vi "Multiple Event Registration1.vi"(11 "Test Case In":refnum<class "Tests Event MessengerM.lvclass">) -> (0 "error out":errorcluster, 3 "Test Case Out":refnum<class "Tests Event MessengerM.lvclass">)   [LabVIEW 2020, in "Tests Event MessengerM.lvclass"]
uses:
  Tests Event MessengerM.lvclass
  C:/Program Files/National Instruments/LabVIEW 2026/vi.lib/Astemes/LUnit/Test Case.lvclass
  <vilib>/Astemes/LUnit/Test Case.lvclass/Test Case.ctl
  4993e8ee-a06a-463a-9684-69129f64d5ce.vi
  f83728eb-1bcd-4ed9-8e7f-64fc7c525065.vi
  f08c0817-9d14-46ec-b6fc-521ef44bde51.vi
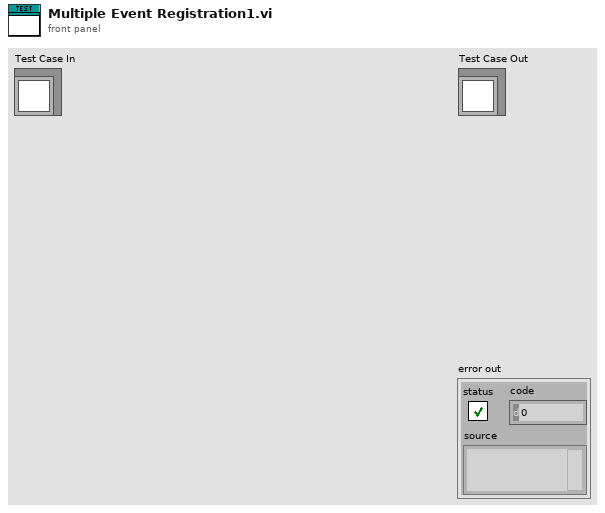
[diagram p1: front panel]
types:
  T1 = typedef "Event MessengerM-bool.lvlib/))Channel.ctl" = refnum<queue>
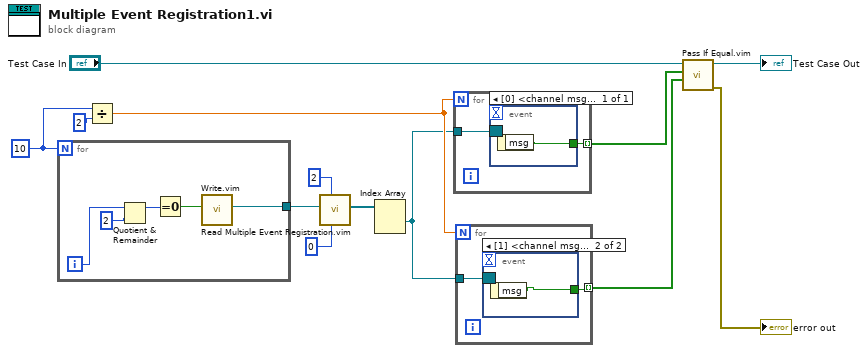
[diagram p0: block diagram]
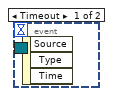
[diagram p2: hidden frame]
diagram:
  w8 = 10
  n1 = for {
    N: w8 -> [_]
    tunnel: [w15] -> w10
    i -> [w18]
    n2 = Quotient & Remainder(x=w18, y=2) -> (x-y*floor(x/y)=w17:i32)  [unwired: 1 out]
    n3 = Equal To 0?(x=w17) -> (x = 0?=w16:bool)
    n4 = call "Write.vim"("element"=w16) -> ("channel"=w15:T1)  [unwired: 9 in, 1 out]
  }
  n5 = Divide(x=w8, y=2) -> (x/y=w6:dbl)
  n6 = call "Read Multiple Event Registration.vim"("subchannel"=0, "number of event structures"=u16 2, "channel in"=w10) -> ("event registration refnums"=w5:refnum<event-registration>[])  [unwired: 8 in]
  n7 = Index Array(array=w5) -> (element #1=w4:refnum<event-registration>)  [unwired: 2 in, 1 out]
  n8 = for {
    N: w6 -> [_]
    tunnel: w4 -> [w20]
    tunnel: [w19] -> w2 mode=indexing
    n9 = event shown="[0] <channel msg>: User Event" {
      selector: w20 -> [_]
      dyn-events: _ -> [_]
      timeout: _ -> [_]
      tunnel: [w21] -> w19
      event User Event {
        n10 = event-data() -> ("msg"=w21:bool)  [unwired: 1 in]
      }
    }
  }
  n11 = for {
    N: w6 -> [_]
    tunnel: w4 -> [w23]
    tunnel: [w22] -> w3 mode=indexing
    n12 = event shown="[1] <channel msg>: User Event" {
      selector: w23 -> [_ _]
      dyn-events: _ -> [_ _]
      timeout: _ -> [_ _]
      tunnel: [_ w24] -> w22
      event Timeout {
        n13 = event-data() -> ()  [unwired: 1 in, 3 out]
      }
      event User Event {
        n14 = event-data() -> ("msg"=w24:bool)  [unwired: 1 in]
      }
    }
  }
  n15 = call "Pass If Equal.vim"("Actual"=w3, "Expected"=w2, "LUnit Test Case In"="Test Case In") -> ("error out"=→"error out":errorcluster, "LUnit Test Case Out"=→"Test Case Out":refnum<class "Tests Event MessengerM.lvclass">)  [unwired: 7 in]
